vi "NetWeave.vi"(0 "Length":dbl, 1 "Spacing":dbl, 2 "LineNo":i32, 3 "error in":errorcluster, 4 "MinJT":dbl, 5 "Vel":dbl, 6 "MaxJT":dbl, 7 "StartPos":dbl[](array[numeric]), 8 "Acc":dbl, 9 "LayerNo":i32) -> (10 "error out":errorcluster)   [LabVIEW 2022 SP3]
uses:
  Global 3.vi
  Newport.XPS.CommandInterface
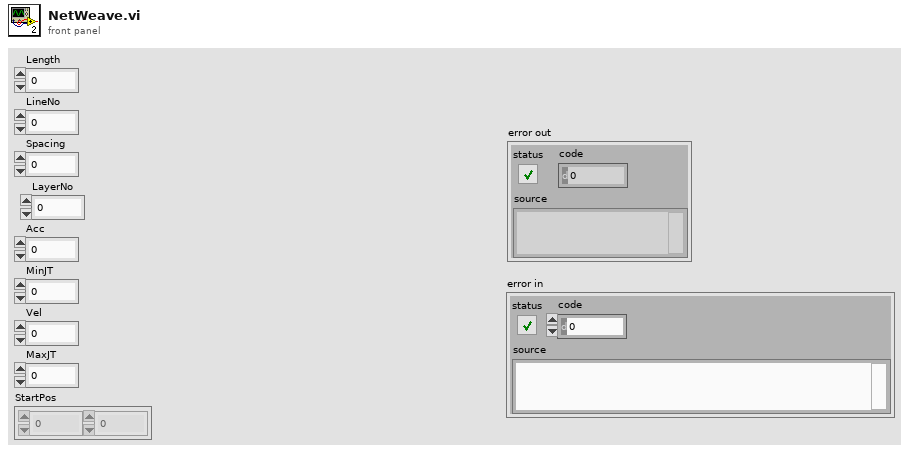
[diagram p1: front panel]
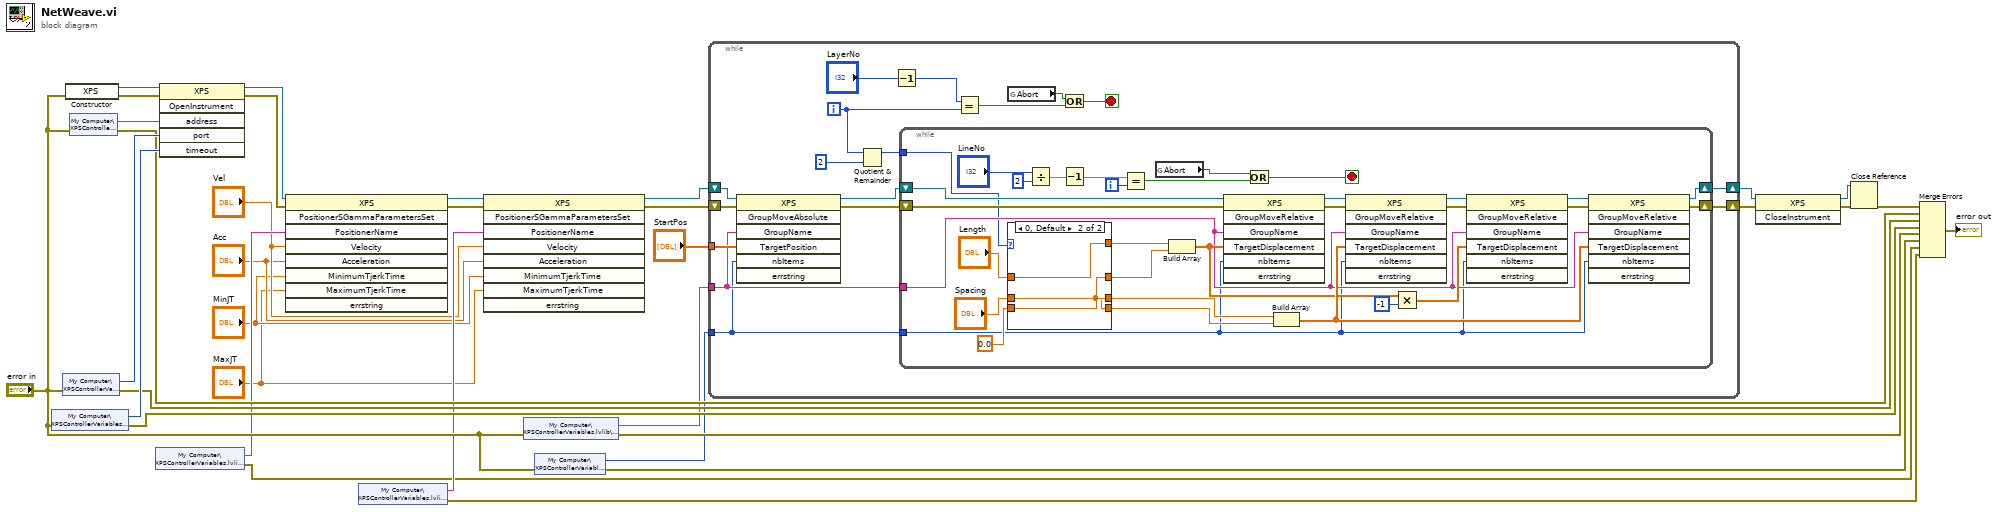
[diagram p0: block diagram]
diagram:
  n1 = shared-variable "My Computer\\XPSControllerVariables.lvlib\\Timeout"(error in="error in") -> (w30:i16, error out=w25:errorcluster)
  n2 = shared-variable "My Computer\\XPSControllerVariables.lvlib\\Port"(error in="error in") -> (w31:i16, error out=w26:errorcluster)
  n3 = constructor class="XPS"(error in="error in") -> (reference out=w34:refnum<k24>, error out=w33:errorcluster)  [unwired: 2 in, 1 out]
  n4 = shared-variable "My Computer\\XPSControllerVariables.lvlib\\IP"(error in="error in") -> (w32:string, error out=w27:errorcluster)
  n5 = shared-variable "My Computer\\XPSControllerVariables.lvlib\\PosNameX"() -> (w13:string, error out=w6:errorcluster)  [unwired: 1 in]
  n6 = invoke class="XPS" method="OpenInstrument"(reference=w34, error in=w33, "address"=w32, "port"=w31, "timeout"=w30) -> (reference out=w19:refnum<k24>, error out=w18:errorcluster)  [unwired: 1 in, 4 out]
  n7 = invoke class="XPS" method="PositionerSGammaParametersSet"(reference=w19, error in=w18, "PositionerName"=w13, "Velocity"="Vel", "Acceleration"="Acc", "MinimumTjerkTime"="MinJT", "MaximumTjerkTime"="MaxJT") -> (reference out=w17:refnum<k24>, error out=w16:errorcluster)  [unwired: 2 in, 7 out]
  n8 = shared-variable "My Computer\\XPSControllerVariables.lvlib\\PosNameY"() -> (w12:string, error out=w5:errorcluster)  [unwired: 1 in]
  n9 = invoke class="XPS" method="PositionerSGammaParametersSet"(reference=w17, error in=w16, "PositionerName"=w12, "Velocity"="Vel", "Acceleration"="Acc", "MinimumTjerkTime"="MinJT", "MaximumTjerkTime"="MaxJT") -> (reference out=w15:refnum<k24>, error out=w14:errorcluster)  [unwired: 2 in, 7 out]
  n10 = shared-variable "My Computer\\XPSControllerVariables.lvlib\\GroupName"(error in="error in") -> (w2:string, error out=w24:errorcluster)
  n11 = shared-variable "My Computer\\XPSControllerVariables.lvlib\\nbitem"(error in="error in") -> (w1:i16, error out=w20:errorcluster)
  n12 = while {
    tunnel: "StartPos" -> [w49]
    tunnel: w2 -> [w44]
    tunnel: w1 -> [w43]
    shift-right: [w46] -> w4
    shift-left: w15 -> [w51]
    shift-right: [w45] -> w3
    shift-left: w14 -> [w50]
    i -> [w37]
    stop <- w40 stop-if-true
    n13 = invoke class="XPS" method="GroupMoveAbsolute"(reference=w51, error in=w50, "GroupName"=w44, "TargetPosition"=w49, "nbItems"=w43) -> (reference out=w48:refnum<k24>, error out=w47:errorcluster)  [unwired: 2 in, 5 out]
    n14 = Quotient & Remainder(x=w37, y=2) -> (x-y*floor(x/y)=w38:i32)  [unwired: 1 out]
    n15 = Decrement(x="LayerNo") -> (x-1=w35:i32)
    n16 = while {
      tunnel: w44 -> [w57]
      tunnel: w43 -> [w56]
      shift-right: [w63] -> w46
      shift-left: w48 -> [w83]
      shift-right: [w62] -> w45
      shift-left: w47 -> [w82]
      tunnel: w38 -> [w52]
      i -> [w78]
      stop <- w75 stop-if-true
      n17 = case shown="0, Default" w52 {
        tunnel: [w85 w89] -> w74
        tunnel: "Length" -> [w86 w89]
        tunnel: [w86 w88] -> w72
        tunnel: 0.0 -> [w85 w88]
        tunnel: [w84 w88] -> w70
        tunnel: [w85 w87] -> w69
        tunnel: "Spacing" -> [w84 w87]
        frame 1 {
        }
        frame 0, Default {
        }
      }
      n18 = Divide(x="LineNo", y=2) -> (x/y=w53:dbl)
      n19 = Decrement(x=w53) -> (x-1=w79:dbl)
      n20 = Equal?(x=w79, y=w78) -> (x = y?=w76:bool)
      n21 = global read "Global 3.vi" "Abort"() -> (w77:bool)
      n22 = Build Array(w74, w72) -> (w60:dbl[])
      n23 = invoke class="XPS" method="GroupMoveRelative"(reference=w83, error in=w82, "GroupName"=w57, "TargetDisplacement"=w60, "nbItems"=w56) -> (reference out=w81:refnum<k24>, error out=w80:errorcluster)  [unwired: 2 in, 5 out]
      n24 = Or(x=w77, y=w76) -> (x .or. y?=w75:bool)
      n25 = Build Array(w70, w69) -> (w61:dbl[])
      n26 = invoke class="XPS" method="GroupMoveRelative"(reference=w81, error in=w80, "GroupName"=w57, "TargetDisplacement"=w61, "nbItems"=w56) -> (reference out=w67:refnum<k24>, error out=w66:errorcluster)  [unwired: 2 in, 5 out]
      n27 = Multiply(x=w60, y=-1) -> (x*y=w58:dbl[])
      n28 = invoke class="XPS" method="GroupMoveRelative"(reference=w67, error in=w66, "GroupName"=w57, "TargetDisplacement"=w58, "nbItems"=w56) -> (reference out=w65:refnum<k24>, error out=w64:errorcluster)  [unwired: 2 in, 5 out]
      n29 = invoke class="XPS" method="GroupMoveRelative"(reference=w65, error in=w64, "GroupName"=w57, "TargetDisplacement"=w61, "nbItems"=w56) -> (reference out=w63:refnum<k24>, error out=w62:errorcluster)  [unwired: 2 in, 5 out]
    }
    n30 = Equal?(x=w35, y=w37) -> (x = y?=w41:bool)
    n31 = global read "Global 3.vi" "Abort"() -> (w42:bool)
    n32 = Or(x=w42, y=w41) -> (x .or. y?=w40:bool)
  }
  n33 = invoke class="XPS" method="CloseInstrument"(reference=w4, error in=w3) -> (reference out=w29:refnum<k24>, error out=w28:errorcluster)  [unwired: 1 in, 1 out]
  n34 = Close Reference(reference=w29, error in (no error)=w28) -> (error out=w23:errorcluster)
  n35 = Merge Errors(w23, w27, w26, w25, w24, w20, w6, w5) -> (→"error out":errorcluster)
